vi "Export.vi"(8 "error in (no error)":errorcluster, 9 "Selected GObjects Only? (F)":bool, 10 "VI Snippet Path (.png)":path, 11 "VI Refnum":refnum<vi>) -> (0 "error out":errorcluster, 3 "dup VI Refnum":refnum<vi>)   [LabVIEW 2022 SP3, in "VI-Snippet.lvlib"]
doc: "Exports a VI Snippet to the <b>VI Snippet Path (.png)</b> specified and embeds the <b>VI Refnum</b> content. If <b>Selected GObjects Only?</b> is True, this exports the currently selected block diagram objects. Otherwise this exports the entire VI."
uses:
  VI-Snippet.lvlib
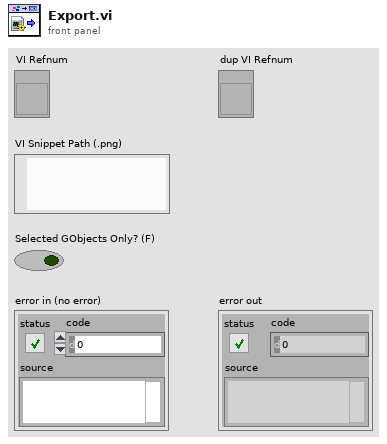
[diagram p1: front panel]
types:
  T1 = typedef "VI-Snippet.lvlib/Snippet.ctl" = cluster{"Image":cluster{"image type":i32, "image depth":i32, "image":u8[], "mask":u8[], "colors":u32[], "Rectangle":cluster{"left":i16, "top":i16, "right":i16, "bottom":i16}}, "niVI":string}
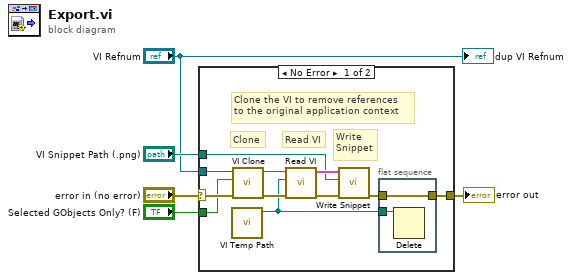
[diagram p0: block diagram]
diagram:
  n1 = case shown="No Error" "error in (no error)" {
    selector: "error in (no error)" -> [w15 w19]
    tunnel: "VI Snippet Path (.png)" -> [w7 _]
    tunnel: [w16 w19] -> w3
    tunnel: "VI Refnum" -> [w14 _]
    tunnel: "Selected GObjects Only? (F)" -> [w13 _]
    frame No Error {
      # "Clone the VI to remove references\nto the original application context"
      # "Read VI"
      # "Clone"
      # "Write\nSnippet"
      n2 = call "VI Temp Path.vi"() -> ("Path (.vi)"=w10:path)  [unwired: 11 in]
      n3 = call "VI Clone.vi"("error in (no error)"=w15, "Selected GObjects Only? (F)"=w13, "Original VI Refnum"=w14) -> ("error out"=w12:errorcluster, "Cloned VI Refnum"=w11:refnum<vi>)  [unwired: 7 in]
      n4 = call "Read VI.vi"("error in (no error)"=w12, "VI Path (.vi)"=w10, "VI Refnum"=w11) -> ("error out"=w9:errorcluster, "Snippet"=w8:T1)  [unwired: 7 in]
      n5 = call "Write Snippet.vi"("error in (no error)"=w9, "VI Snippet (.png)"=w7, "Snippet"=w8) -> ("error out"=w6:errorcluster)  [unwired: 8 in]
      n6 = flat-sequence {
        tunnel: w10 -> [w18]
        tunnel: [w17] -> w16
        tunnel: w6 -> [w17]
        frame #0 {
          n7 = Delete(path (use dialog)=w18) -> ()  [unwired: 4 in, 3 out]
        }
      }
    }
    frame Error {
    }
  }
  "error out" <- w3
  "dup VI Refnum" <- "VI Refnum"
